vi "PerformStack.vi"() -> ()   [LabVIEW 2010]
uses:
  Serial Controller.lvclass
panel:
  in  "VISA resource name":refnum<visa-resource-name>="COM3"
  out "AllPositions":dbl[][](array[numeric])
  in  "Reset first":bool
  out "Steps done":i32
  in  "Steps":i32=30
  in  "Delay (ms)":u32=10000
  in  "Delta":dbl[](array[numeric])=[0.0, 0.0, 5.0]
  in  "stop":bool
  out "error out":errorcluster
  out "Position":dbl[](array[numeric])
  out "Firmware Version":u16
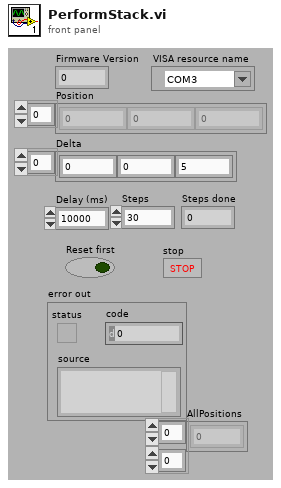
[diagram p1: front panel]
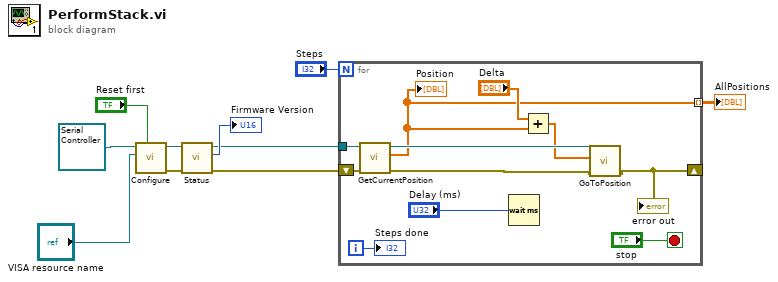
[diagram p0: block diagram]
diagram:
  n1 = call-dynamic "Configure.vi"("Reset"="Reset first", "VISA resource name"="VISA resource name", "Serial Controller in"=refnum<class "Serial Controller.lvclass"> refnum ("Serial Controller.lvclass")) -> ("error out"=w4:errorcluster, "Serial Controller out"=w5:refnum<class "Serial Controller.lvclass">)  [unwired: 7 in]
  n2 = call-dynamic "Status.vi"("error in (no error)"=w4, "Serial Controller in"=w5) -> ("error out"=w8:errorcluster, "Firmware Version"=→"Firmware Version":u16, "Serial Controller out"=w9:refnum<class "Serial Controller.lvclass">)  [unwired: 7 in]
  n3 = for {
    N: "Steps" -> [_]
    tunnel: w9 -> [w21]
    shift-right: [w16] -> _
    shift-left: w8 -> [w20]
    tunnel: [w11] -> w2 mode=indexing
    i -> [w12]
    stop <- "stop" stop-if-true
    n4 = call-dynamic "GetCurrentPosition.vi"("error in (no error)"=w20, "Serial Controller in"=w21) -> ("error out"=w18:errorcluster, "Position"=w11:dbl[], "Serial Controller out"=w17:refnum<class "Serial Controller.lvclass">)  [unwired: 7 in]
    "Position" <- w11
    n5 = Wait (ms)(milliseconds to wait="Delay (ms)") -> ()  [unwired: 1 out]
    n6 = Add(x="Delta", y=w11) -> (x+y=w14:dbl[])
    n7 = call-dynamic "GoToPosition.vi"("error in (no error)"=w18, "Position"=w14, "Serial Controller in"=w17) -> ("error out"=w16:errorcluster)  [unwired: 7 in, 1 out]
    "error out" <- w16
    "Steps done" <- w12
  }
  "AllPositions" <- w2
